vi "Hoop align with x value.vi"(0 "Current X":dbl, 5 "SetPoint X":dbl=160.0) -> (4 "motor values":cluster{"Left Motor":dbl, "Right Motor":dbl}, 6 "Aligned?":bool)   [LabVIEW 2011]
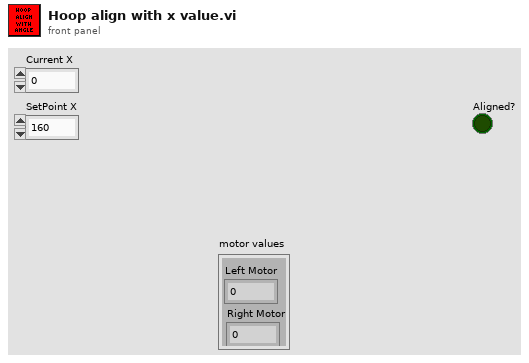
[diagram p1: front panel]
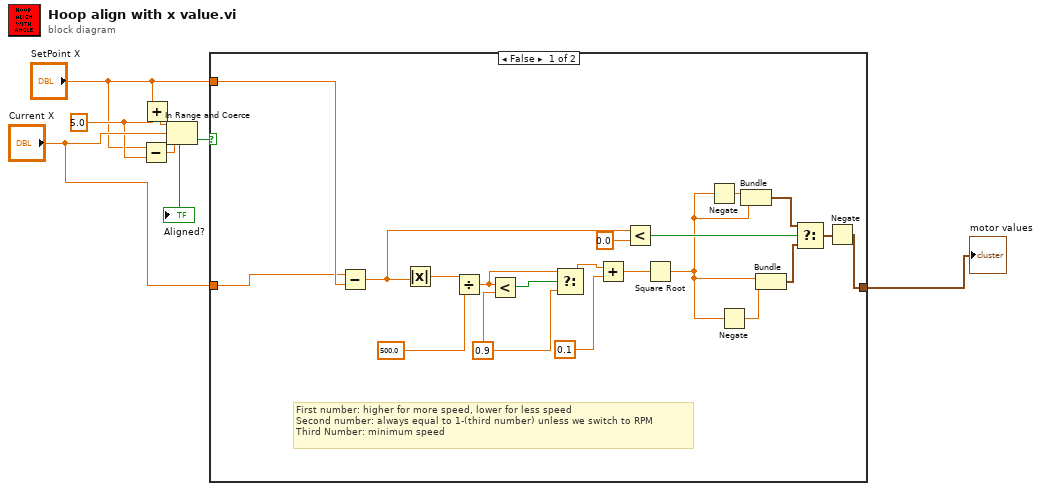
[diagram p0: block diagram]
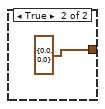
[diagram p2: hidden frame]
diagram:
  w3 = 5.0 ("y")
  n1 = Subtract(x="SetPoint X", y=w3) -> (x-y=w2:dbl)
  n2 = Add(x="SetPoint X", y=w3) -> (x+y=w4:dbl)
  n3 = In Range and Coerce(upper limit=w4, x="Current X", lower limit=w2) -> (In Range?=w6:bool)  [unwired: 1 out]
  "Aligned?" <- w6
  n4 = case shown="False" w6 {
    tunnel: [w8 cluster{"Left Motor":dbl, "Right Motor":dbl} {"Left Motor"=0.0, "Right Motor"=0.0} ("motor values")] -> w7
    tunnel: "Current X" -> [w9 _]
    tunnel: "SetPoint X" -> [w20 _]
    frame False {
      w24 = 0.9 ("y")
      # "First number: higher for more speed, lower for less speed\nSecond number: always equal to 1-(third number) unless we switch to RPM\nThird Number: minimum speed"
      n5 = Subtract(x=w9, y=w20) -> (x-y=w19:dbl)
      n6 = Absolute Value(x=w19) -> (abs(x)=w22:dbl)
      n7 = Divide(x=w22, y=500.0) -> (x/y=w21:dbl)
      n8 = Less?(x=w21, y=w24) -> (x < y?=w25:bool)
      n9 = Select(t=w21, s=w25, f=w24) -> (s? t:f=w23:dbl)
      n10 = Add(x=w23, y=0.1) -> (x+y=w11:dbl)
      n11 = Less?(x=w19, y=0.0) -> (x < y?=w17:bool)
      n12 = Square Root(x=w11) -> (sqrt(x)=w10:dbl)
      n13 = Negate(x=w10) -> (-x=w13:dbl)
      n14 = Negate(x=w10) -> (-x=w12:dbl)
      n15 = Bundle(w13, w10) -> (w16:cluster{dbl, dbl})  [unwired: 1 in]
      n16 = Bundle(w10, w12) -> (w15:cluster{dbl, dbl})  [unwired: 1 in]
      n17 = Select(t=w16, s=w17, f=w15) -> (s? t:f=w14:cluster{dbl, dbl})
      n18 = Negate(x=w14) -> (-x=w8:cluster{dbl, dbl})
    }
    frame True {
    }
  }
  "motor values" <- w7
